vi "Database Lock.vi"(8 "error in (no error)":errorcluster, 9 "Requesting Module":T1, 11 "Status":T2) -> (0 "error out":errorcluster, 3 "Status":T2)   [LabVIEW 2016]
doc: "Lock access to the database"
uses:
  Controls/Database Status.ctl
  Architecture/Message Queue/Message Cluster.ctl
  Car Wash Controller/Controls/Steps.ctl
  Car Wash Controller/Controls/Stations.ctl
  Architecture/Modules.ctl
  Architecture/Message Queue/Message Queue.lvlib
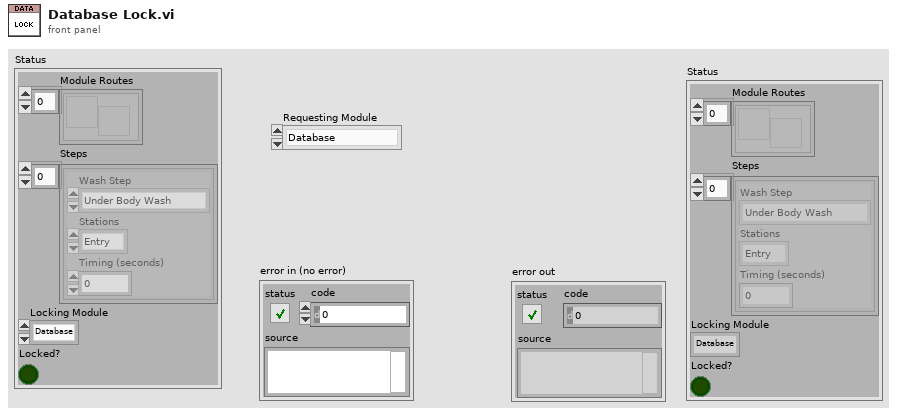
[diagram p1: front panel]
types:
  T1 = typedef "Modules.ctl" = enum16{"Database", "Car Wash Controller", "Console"}
  T2 = typedef "Database Status.ctl" = cluster{"Module Routes":refnum<user-event>[], "Steps":cluster{"Wash Step":T3, "Stations":T4, "Timing (seconds)":u32}[], "Locking Module":T1, "Locked?":bool}
  T3 = typedef "Steps.ctl" = enum16{"Under Body Wash", "Bug Remover", "Pre-Soak", "High Pressure Wash", "Low Pressure Wax", "Spot Free Rinse", "Tire Shine Foam", "Air Dry"}
  T4 = typedef "Stations.ctl" = enum16{"Entry", "Station 1", "Station 2", "Station 3", "Exit"}
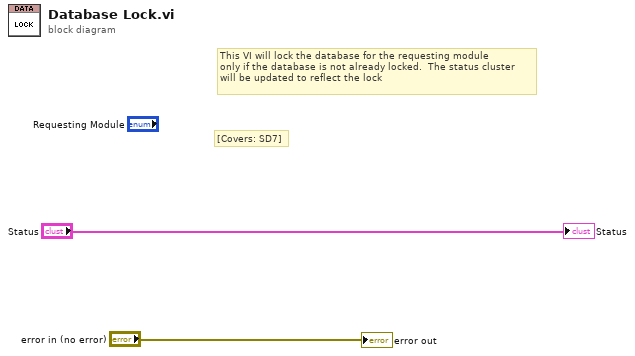
[diagram p0: block diagram]
diagram:
  # "[Covers: SD7]"
  # "This VI will lock the database for the requesting module\nonly if the database is not already locked.  The status cluster\nwill be updated to reflect the lock"
  "error out" <- "error in (no error)"
  "Status" <- "Status"
